vi "Remove Data Replay Offset RTM Dependency.vi"(8 "error in (no error)":errorcluster, 9 "Menu hierarchy in":string[](array[string]), 11 "Node Ptr":u64 format="%.0x") -> (0 "error out":errorcluster, 1 "Menu hierarchy out":string[](array[string]), 3 "Action":T1)   [LabVIEW 2011, in "Engine Sim System Explorer.lvlib"]
uses:
  Engine Sim System Explorer.lvlib
  <vilib>/NI Veristand/Custom Device API/Custom Device RTM Dependency.ctl
  Shared/Engine Simulation Global.vi
  <vilib>/NI Veristand/Custom Device Tools/Custom Device Utility Library/NI VeriStand - Search for Item by Name.vi
  <vilib>/NI Veristand/Custom Device API/Get Item Property (Boolean).vi
  <vilib>/NI Veristand/Custom Device API/Custom Device API.lvlib
  Engine Simulation Shared.lvlib
  <vilib>/NI Veristand/Custom Device Tools/Custom Device Utility Library/Custom Device Utility Library.lvlib
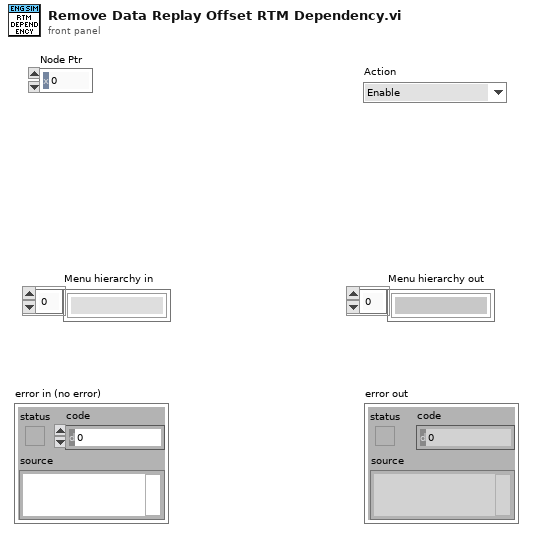
[diagram p1: front panel]
types:
  T1 = typedef "Custom Device API.lvlib/Custom Device RTM Dependency.ctl" = enum16{"Enable", "Disable", "Hide"}
  T2 = typedef "Custom Device API.lvlib/Custom Device Item Ref.ctl" = u64
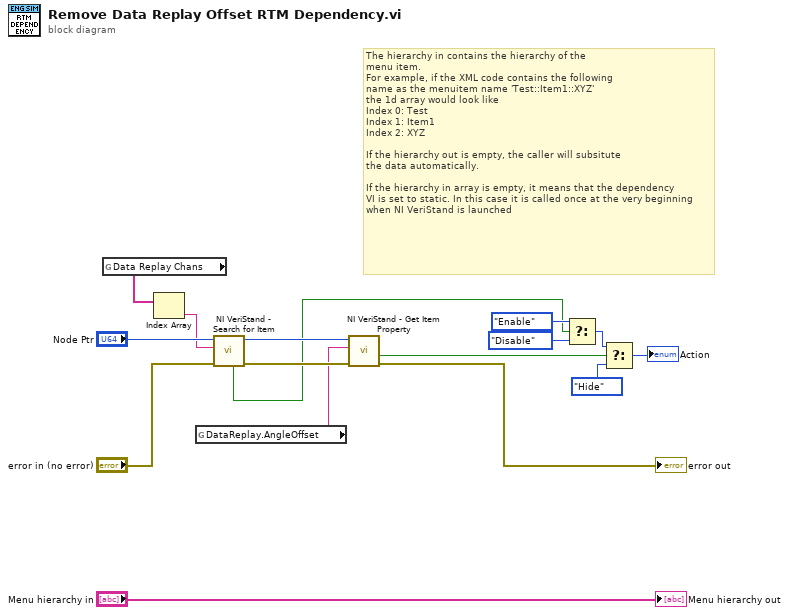
[diagram p0: block diagram]
diagram:
  # "The hierarchy in contains the hierarchy of the\nmenu item.\nFor example, if the XML code contains the following\nname as the menuitem name 'Test::Item1::XYZ'\nthe 1d array would look like\nIndex 0: Test\nIndex 1: Item1\nIndex 2: XYZ\n\nIf the hierarchy out is empty, the caller will subsitute\nthe data automatically.\n\nIf the hierarchy in array is empty, it means that the dependency\nVI is set to static. In this case it is called once at the very beginning\nwhen NI VeriStand is launched"
  n1 = global read "Engine Simulation Global.vi" "Data Replay Chans"() -> (w3:string[])
  n2 = Index Array(array=w3) -> (element=w2:string)  [unwired: 1 in]
  n3 = global read "Engine Simulation Global.vi" "DataReplay.AngleOffset"() -> (w4:string)
  n4 = call-poly <vilib>:"NI VeriStand - Search for Item.vi"("error in"="error in (no error)", "Item Name"=w2, "Section Ref in"="Node Ptr") -> ("error out"=w15:errorcluster, "Section Ref out"=w16:T2, "Found"=w1:bool)  [unwired: 5 in, 1 out]
  n5 = call-poly <vilib>:"NI VeriStand - Get Item Property.vi"("error in (no error)"=w15, "Property Name"=w4, "Item Ref in"=w16) -> ("error out"=→"error out":errorcluster, "Value"=w9:bool)  [unwired: 5 in, 2 out]
  n6 = Select(t=Custom_Device_RTM_Dependency."Enable" ("Action"), s=w1, f=Custom_Device_RTM_Dependency."Disable") -> (s? t:f=w8:T1)
  n7 = Select(t=w8, s=w9, f=Custom_Device_RTM_Dependency."Hide" ("Action")) -> (s? t:f=→"Action":T1)
  "Menu hierarchy out" <- "Menu hierarchy in"
